vi "MB Serial Example Master MK2.vi"() -> ()   [LabVIEW 2021]
uses:
  API/Wrapper/API Main.lvlib
  API/Master/Modbus Master.lvclass
  API/Wrapper/Create Serial Master.vi
  Data Model/Identification Parameters.ctl
  Data Model/Device Data Model.lvclass
  Master Function Definition/Read Device ID code.ctl
panel:
  in  "VISA resource name":refnum<visa-resource-name>="COM7"
  out "loop time":dbl
  in  "Read Device ID code":T1
  in  "Object ID":u8
  out "Objects":T2[](array[typedef]) {"Object ID" format="%x"}
  out "exception status":u8
  out "discrete inputs":bool[](array[boolean])
  out "Input Registers":u16[](array[numeric])=[0, 0, 2, 2]
  out "error out":errorcluster
  out "Holding Registers":u16[](array[numeric])=[0, 0, 2, 2]
  in  "Write Single Register":u16[](array[numeric])=[0, 0, 2, 2]
  in  "Write Multiple Registers":cluster{"Set Registers":bool, u16[]}={"Set Registers"=FALSE, [0, 0, 2, 2]}
  in  "Write Multiple Coils":T3={"Write Single Coils 2"=[TRUE, FALSE, FALSE, TRUE], "Set Coils"=FALSE}
  in  "Write Single Coils":bool[](array[boolean])=[FALSE, FALSE, FALSE, FALSE] caption="Coils to Write"
  in  "Stop":bool
  out "Coils":bool[](array[boolean])=[TRUE, FALSE, FALSE, TRUE] caption="Slave Discrete Inputs"
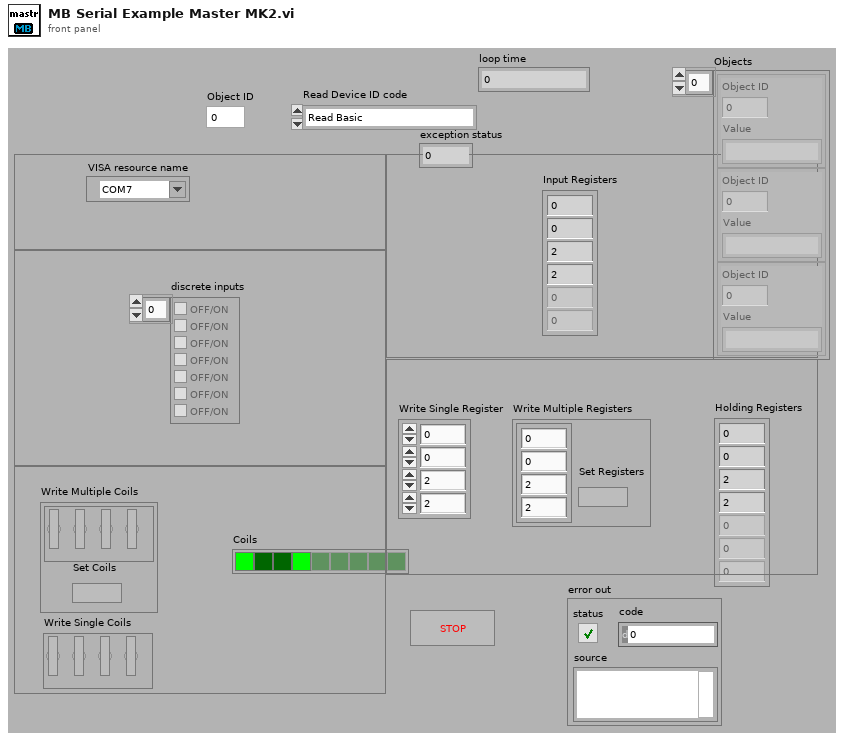
[diagram p1: front panel]
types:
  T1 = typedef "Device Data Model.lvclass/Read Device ID code.ctl" = enum8{"Read Basic", "Read Regular", "Read Extended", "Read Specific"}
  T2 = typedef "Device Data Model.lvclass/Identification Parameters.ctl" = cluster{"Object ID":u8, "Value":string}
  T3 = cluster{"Write Single Coils 2":bool[], "Set Coils":bool}
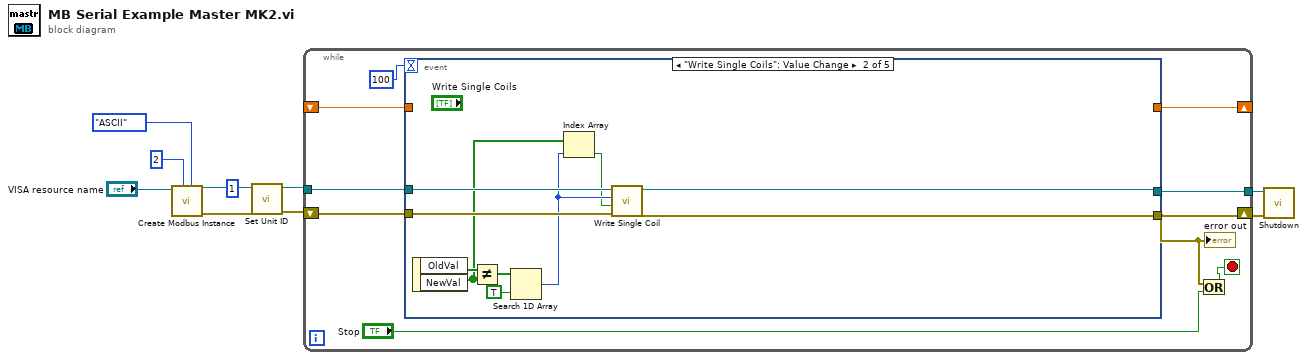
[diagram p0: block diagram]
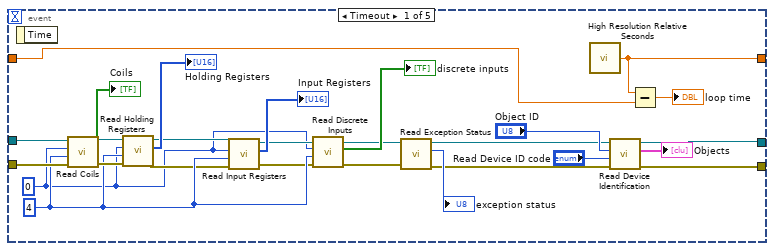
[diagram p2: hidden frame]
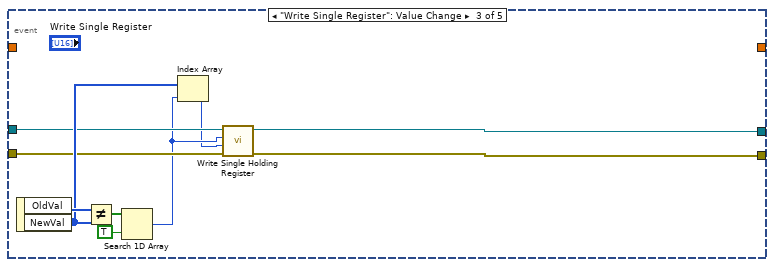
[diagram p3: hidden frame]
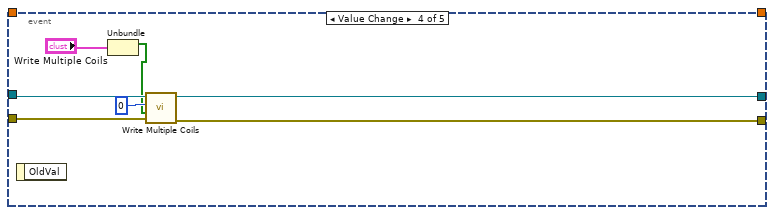
[diagram p4: hidden frame]
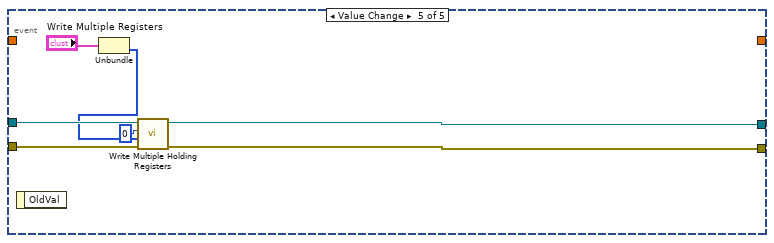
[diagram p5: hidden frame]
diagram:
  n1 = call-poly "Create Modbus Instance.vi"("serial type"=enum16{"RTU", "ASCII"}."ASCII" ("Serial Type"), "unit ID"=u8 2 ("Unit ID"), "VISA resource name"="VISA resource name") -> ("error out"=w3:errorcluster, "serial master instance"=w4:refnum<class "Modbus Master.lvclass">)  [unwired: 7 in]
  n2 = call "Set Unit ID.vi"("error in (no error)"=w3, "unit ID"=u8 1 ("Unit ID"), "Modbus master in"=w4) -> ("error out"=w6:errorcluster, "Modbus master out"=w5:refnum<class "Modbus Master.lvclass">)  [unwired: 7 in]
  n3 = while {
    tunnel: w5 -> [w18]
    tunnel: [w17] -> w9
    shift-right: [w13] -> w10
    shift-left: w6 -> [w16]
    shift-right: [w15] -> _
    shift-left: _ -> [w14]
    stop <- w11 stop-if-true
    n4 = event shown="[1] \"Write Single Coils\": Value Change" {
      selector: _ -> [_ _ _ _ _]
      dyn-events: _ -> [_ _ _ _ _]
      timeout: 100 -> [_ _ _ _ _]
      tunnel: [w23 w54 w62 w69 w76] -> w13
      tunnel: w18 -> [w46 w56 w60 w72 w78]
      tunnel: [w25 w53 w61 w68 w77] -> w17
      tunnel: w16 -> [w45 w55 w59 w71 w79]
      tunnel: [w22 _ _ _ _] -> w15
      tunnel: w14 -> [w21 _ _ _ _]
      event Timeout {
        w39 = u16 4 ("Number of coils")
        w32 = u16 0 ("Starting Address")
        n5 = event-data() -> ()  [unwired: 2 out]
        n6 = call-dynamic "Read Coils.vi"("error in (no error)"=w45, "number of coils"=w39, "starting address"=w32, "Modbus master in"=w46) -> ("error out"=w42:errorcluster, "coil values"=→"Coils":bool[], "Modbus master out"=w43:refnum<class "Modbus Master.lvclass">)  [unwired: 5 in]
        n7 = call-dynamic "Read Holding Registers.vi"("error in (no error)"=w42, "number of holding registers"=w39, "starting address"=w32, "Modbus master in"=w43) -> ("error out"=w35:errorcluster, "register values"=→"Holding Registers":u16[], "Modbus master out"=w36:refnum<class "Modbus Master.lvclass">)  [unwired: 5 in]
        n8 = call-dynamic "Read Input Registers.vi"("error in (no error)"=w35, "number of input registers"=w39, "starting address"=w32, "Modbus master in"=w36) -> ("error out"=w33:errorcluster, "register values"=→"Input Registers":u16[], "Modbus master out"=w34:refnum<class "Modbus Master.lvclass">)  [unwired: 5 in]
        n9 = call-dynamic "Read Discrete Inputs.vi"("error in (no error)"=w33, "number of discrete inputs"=w39, "starting address"=w32, "Modbus master in"=w34) -> ("error out"=w30:errorcluster, "discrete input values"=→"discrete inputs":bool[], "Modbus master out"=w31:refnum<class "Modbus Master.lvclass">)  [unwired: 5 in]
        n10 = call-dynamic "Read Exception Status.vi"("error in (no error)"=w30, "Modbus master in"=w31) -> ("error out"=w24:errorcluster, "exception status"=→"exception status":u8, "Modbus master out"=w26:refnum<class "Modbus Master.lvclass">)  [unwired: 7 in]
        n11 = call <vilib>:"High Resolution Relative Seconds.vi"() -> ("relative seconds"=w22:dbl)
        n12 = call-dynamic "Read Device Identification.vi"("error in (no error)"=w24, "read device ID code"="Read Device ID code", "object ID"="Object ID", "Modbus master in"=w26) -> ("error out"=w23:errorcluster, "objects"=→"Objects":cluster{"object ID":u8, "value":string}[], "Modbus master out"=w25:refnum<class "Modbus Master.lvclass">)  [unwired: 5 in]
        n13 = Subtract(x=w22, y=w21) -> (x-y=→"loop time":dbl)
      }
      event "Write Single Coils": Value Change {
        n14 = event-data() -> ("OldVal"=w52:bool[], "NewVal"=w49:bool[])  [unwired: 1 out]
        n15 = Not Equal?(x=w52, y=w49) -> (x != y?=w51:bool[])
        n16 = Search 1D Array(1D array=w51, element=TRUE) -> (index of element=w48:i32)  [unwired: 1 in]
        n17 = Index Array(array=w49, index=w48) -> (element=w47:bool)
        n18 = call-dynamic "Write Single Coil.vi"("error in (no error)"=w55, "coil value"=w47, "address"=w48, "Modbus master in"=w56) -> ("error out"=w54:errorcluster, "Modbus master out"=w53:refnum<class "Modbus Master.lvclass">)  [unwired: 6 in]
      }
      event "Write Single Register": Value Change {
        n19 = event-data() -> ("OldVal"=w64:u16[], "NewVal"=w63:u16[])  [unwired: 1 out]
        n20 = Not Equal?(x=w64, y=w63) -> (x != y?=w66:bool[])
        n21 = Search 1D Array(1D array=w66, element=TRUE) -> (index of element=w58:i32)  [unwired: 1 in]
        n22 = Index Array(array=w63, index=w58) -> (element=w57:u16)
        n23 = call-dynamic "Write Single Holding Register.vi"("error in (no error)"=w59, "holding register value"=w57, "address"=w58, "Modbus master in"=w60) -> ("error out"=w62:errorcluster, "Modbus master out"=w61:refnum<class "Modbus Master.lvclass">)  [unwired: 6 in]
      }
      event "Write Multiple Coils.Set Coils": Value Change {
        n24 = event-data() -> ()  [unwired: 2 out]
        n25 = Unbundle("Write Multiple Coils") -> ("Write Single Coils 2"=w67:bool[])  [unwired: 1 out]
        n26 = call-dynamic "Write Multiple Coils.vi"("error in (no error)"=w71, "coil values"=w67, "starting address"=u16 0 ("Starting Address"), "Modbus master in"=w72) -> ("error out"=w69:errorcluster, "Modbus master out"=w68:refnum<class "Modbus Master.lvclass">)  [unwired: 6 in]
      }
      event "Write Multiple Registers.Set Registers": Value Change {
        n27 = event-data() -> ()  [unwired: 2 out]
        n28 = Unbundle("Write Multiple Registers") -> (w74:u16[])  [unwired: 1 out]
        n29 = call-dynamic "Write Multiple Holding Registers.vi"("error in (no error)"=w79, "holding register values"=w74, "starting address"=u16 0 ("Starting Address"), "Modbus master in"=w78) -> ("error out"=w76:errorcluster, "Modbus master out"=w77:refnum<class "Modbus Master.lvclass">)  [unwired: 6 in]
      }
    }
    "error out" <- w13
    n30 = Or(x=w13, y="Stop") -> (x .or. y?=w11:bool)
  }
  n31 = call-dynamic "Shutdown.vi"("error in (no error)"=w10, "Modbus master in"=w9) -> ()  [unwired: 9 in, 1 out]
